vi "rqcBob SPD State Viewer.vi"() -> ()   [LabVIEW 2018]
uses:
  hidSPDLibForLabView/LibVIs/hidSPD Controls/hidSPD Viwer State.ctl
  hidSPDLibForLabView/hidSPDLibForLabView.lvlib
panel:
  out "SPD2 Heatsink T":sgl(graph) caption="Heatsink T"
  out "SPD2 Diod T":sgl(graph) caption="Diod T"
  out "SPD2 Ready":bool caption="Ready"
  out "error out":errorcluster
  in  "Stop":bool
  out "SPD1 Heatsink T":sgl(graph) caption="Heatsink T"
  out "SPD1 Diod T":sgl(graph) caption="Diod T"
  out "SPD1 Ready":bool caption="Ready"
  # "SPD1"
  # "SPD2"
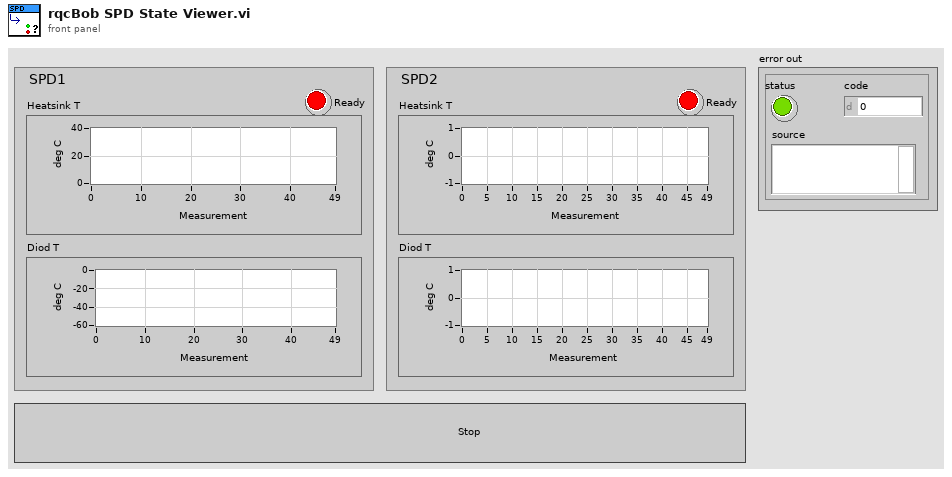
[diagram p1: front panel]
types:
  T1 = typedef "hidSPDLibForLabView.lvlib/hidSPD Viwer State.ctl" = enum16{"open sessions", "close sessions", "read reports"}
  T2 = typedef "hidSPDLibForLabView.lvlib/hidSPD HidDevInfo.ctl" = cluster{"name":string, "path":string}
  T3 = typedef "hidSPDLibForLabView.lvlib/hidSPD Device Session.ctl" = cluster{"spdDevicePointer":u64}
  T4 = typedef "hidSPDLibForLabView.lvlib/hidSPD Simple Report.ctl" = cluster{"Heatsink Temprature":sgl, "Diod Temprature":sgl, "TEC-voltage":sgl, "Diod Bias":sgl, "RF Power":sgl, "Thermal used":sgl, "hv bias used":sgl, "hv code used":u16, "strobe code used":u16, "SPD number":u8, "SPD ready":u8}
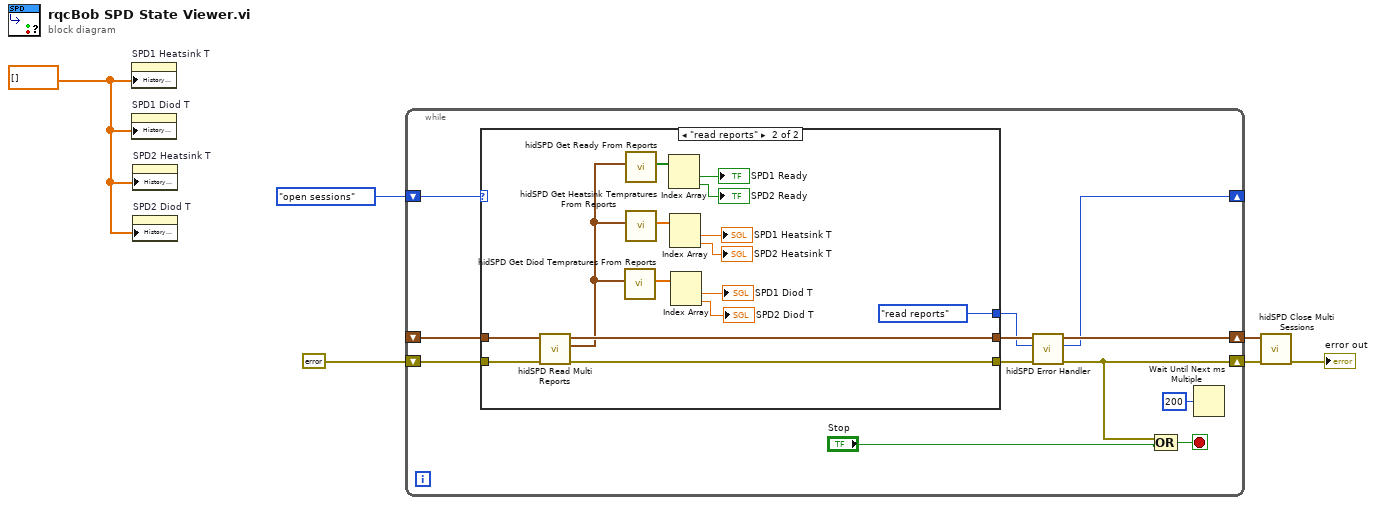
[diagram p0: block diagram]
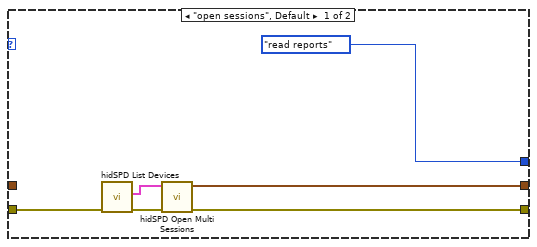
[diagram p2: hidden frame]
diagram:
  w3 = sgl[] [] ("History Data")
  n1 = property on="SPD1 Heatsink T" class="WFChart (strict)"("History Data"=w3) -> ()  [unwired: 2 in, 2 out]
  n2 = property on="SPD1 Diod T" class="WFChart (strict)"("History Data"=w3) -> ()  [unwired: 2 in, 2 out]
  n3 = property on="SPD2 Heatsink T" class="WFChart (strict)"("History Data"=w3) -> ()  [unwired: 2 in, 2 out]
  n4 = property on="SPD2 Diod T" class="WFChart (strict)"("History Data"=w3) -> ()  [unwired: 2 in, 2 out]
  n5 = while {
    shift-right: [w11] -> w5
    shift-left: _ -> [w18]
    shift-right: [w9] -> w4
    shift-left: errorcluster {"status"=FALSE, "code"=0, "source"=""} ("error in (no error)") -> [w17]
    shift-right: [w7] -> _
    shift-left: hidSPD_Viwer_State."open sessions" ("hidSPD Viewer State") -> [w13]
    stop <- w15 stop-if-true
    n6 = case shown="\"read reports\"" w13 {
      tunnel: w18 -> [_ w39]
      tunnel: w17 -> [w20 w38]
      tunnel: [w22 w37] -> w12
      tunnel: [w21 w36] -> w10
      tunnel: [hidSPD_Viwer_State."read reports" ("hidSPD Viewer State") hidSPD_Viwer_State."read reports" ("hidSPD Viewer State")] -> w8
      frame "open sessions", Default {
        n7 = call "hidSPD List Devices.vi"("error in (no error)"=w20) -> ("error out"=w24:errorcluster, "devices list"=w23:T2[])  [unwired: 9 in]
        n8 = call "hidSPD Open Multi Sessions.vi"("error in (no error)"=w24, "devices list"=w23) -> ("error out"=w21:errorcluster, "spdDevSessions out"=w22:T3[])  [unwired: 8 in]
      }
      frame "read reports" {
        n9 = call "hidSPD Read Multi Reports.vi"("error in (no error)"=w38, "spdDevSessions in"=w39) -> ("error out"=w36:errorcluster, "spd Reports"=w35:T4[], "spdDevSessions out"=w37:T3[])  [unwired: 7 in]
        n10 = call "hidSPD Get Diod Tempratures From Reports.vi"("spd Reports in"=w35) -> ("Diod Tempratures"=w32:sgl[])  [unwired: 10 in]
        n11 = call "hidSPD Get Ready From Reports.vi"("spd Reports in"=w35) -> ("Ready"=w30:bool[])  [unwired: 10 in]
        n12 = call "hidSPD Get Heatsink Tempratures From Reports.vi"("spd Reports in"=w35) -> ("Heatsink Tempratures"=w34:sgl[])  [unwired: 10 in]
        n13 = Index Array(array=w30) -> (element #1=→"SPD1 Ready":bool, element #2=→"SPD2 Ready":bool)  [unwired: 2 in]
        n14 = Index Array(array=w34) -> (element #1=→"SPD1 Heatsink T":sgl, element #2=→"SPD2 Heatsink T":sgl)  [unwired: 2 in]
        n15 = Index Array(array=w32) -> (element #1=→"SPD1 Diod T":sgl, element #2=→"SPD2 Diod T":sgl)  [unwired: 2 in]
      }
    }
    n16 = call "hidSPD Error Handler.vi"("error in (no error)"=w10, "hidSPD Viewer State in"=w8, "spdDevSessions in"=w12) -> ("error out"=w9:errorcluster, "hidSPD Viewer State out"=w7:T1, "spdDevSessions out"=w11:T3[])  [unwired: 6 in]
    n17 = Compound Arithmetic op=OR(w9, "Stop") -> (w15:bool)
    n18 = Wait Until Next ms Multiple(millisecond multiple=u32 200) -> ()  [unwired: 1 out]
  }
  n19 = call "hidSPD Close Multi Sessions.vi"("error in (no error)"=w4, "spdDevSessions out"=w5) -> ("error out"=→"error out":errorcluster)  [unwired: 9 in]
